vi "db_plant.id_to_sensors.vi"(6 "plant":u16, 9 "shift reg":u16, 10 "db path":path, 11 "Ring in":refnum<vi>) -> ()   [LabVIEW 2011]
uses:
  DBSqlSelectToArray(1DArrayClusterStringInt).vi
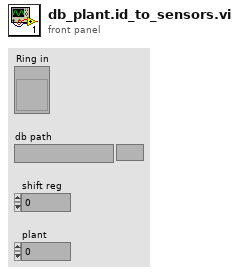
[diagram p1: front panel]
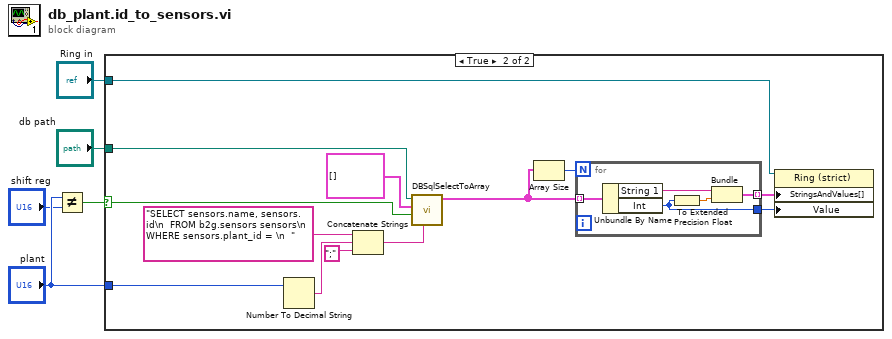
[diagram p0: block diagram]
diagram:
  n1 = Not Equal?(x="plant", y="shift reg") -> (x != y?=w2:bool)
  n2 = case shown="True" w2 {
    selector: w2 -> [_ w12]
    tunnel: "plant" -> [_ w15]
    tunnel: "db path" -> [_ w18]
    tunnel: "Ring in" -> [_ w8]
    frame False {
    }
    frame True {
      n3 = Number To Decimal String(number=w15) -> (decimal integer string=w14:string)  [unwired: 1 in]
      n4 = Concatenate Strings("SELECT sensors.name, sensors.id\n  FROM b2g.sensors sensors\n  WHERE sensors.plant_id = \n  " ("String"), w14, ";" ("string")) -> (w16:string)
      n5 = call-poly "DBSqlSelectToArray.vi"("String"=w16, "enable"=w12, "format"=cluster{"String 1":string, "Int 2":u16}[] [], "connection information"=w18) -> ("shift reg out"=w9:cluster{"String 1":string, "Int":u16}[])  [unwired: 6 in, 1 out]
      n6 = Array Size(array=w9) -> (size(s)=w10:i32)
      n7 = for {
        N: w10 -> [_]
        tunnel: w9 -> [w23] mode=indexing
        tunnel: [w20] -> w7 mode=indexing
        tunnel: [w19] -> w6
        n8 = Unbundle By Name(w23) -> ("String 1"=w21:string, "Int"=w19:u16)
        n9 = To Extended Precision Float(1:w19) -> (0:w22:ext)
        n10 = Bundle("String 1"=w21, w22) -> (w20:cluster{"String 1":string, ext})  [unwired: 1 in]
      }
      n11 = property class="Ring (strict)"(reference=w8, "StringsAndValues[]"=w7, "Value"=w6) -> ()  [unwired: 1 in, 2 out]
    }
  }
